vi "picarx.vi"() -> ()   [LabVIEW 2020]
panel:
  in  "Stop Button":bool
  in  "see  up":bool
  in  "see down":bool
  in  "see right":bool
  in  "see left":bool
  in  "backward":bool
  in  "left":bool
  in  "right":bool
  in  "forward":bool
  in  "stop":bool
  in  "say":bool
  in  "Delay Time (s)":dbl=1.0
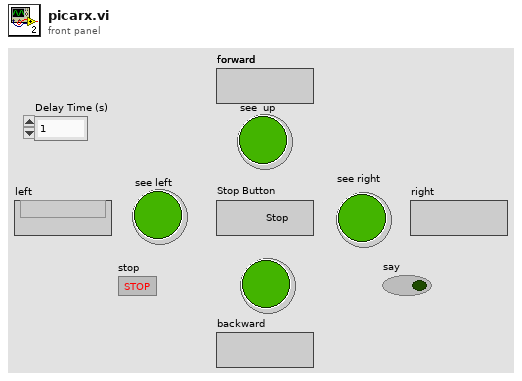
[diagram p1: front panel]
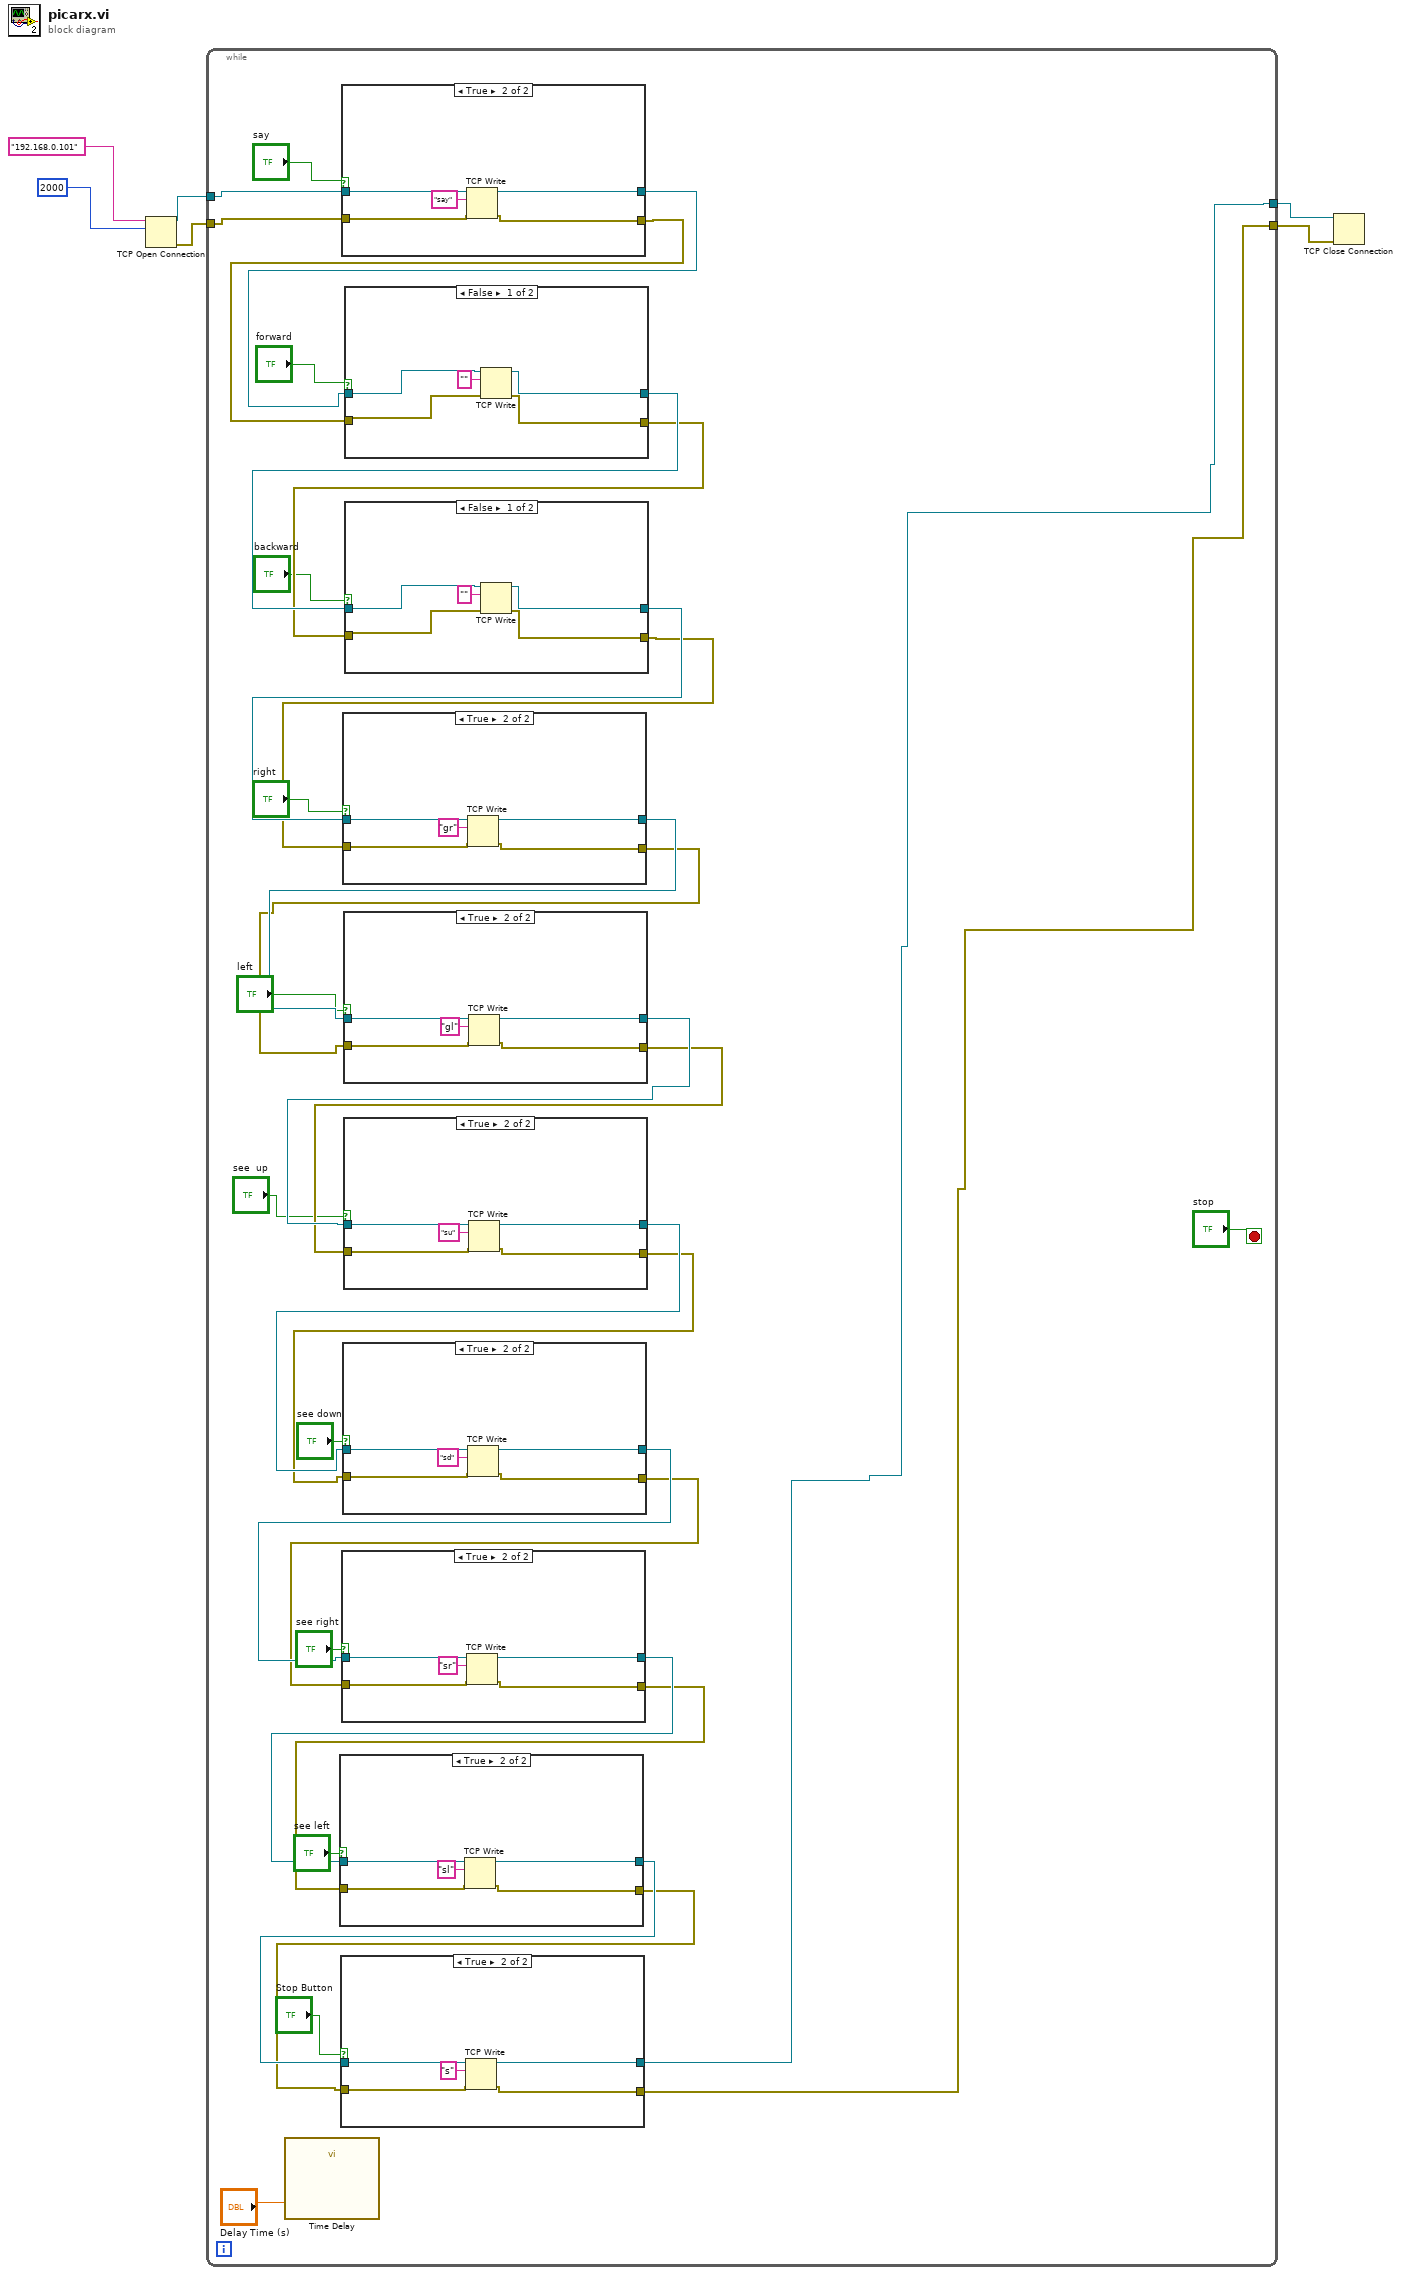
[diagram p0: block diagram]
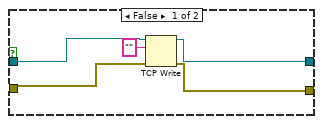
[diagram p2: hidden frame]
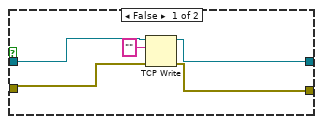
[diagram p3: hidden frame]
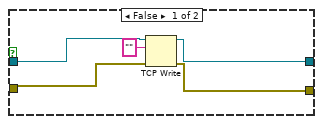
[diagram p4: hidden frame]
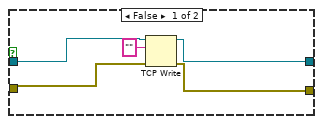
[diagram p5: hidden frame]
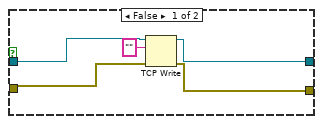
[diagram p6: hidden frame]
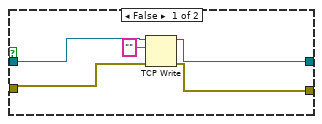
[diagram p7: hidden frame]
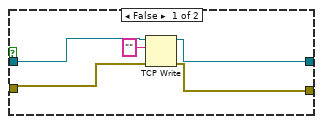
[diagram p8: hidden frame]
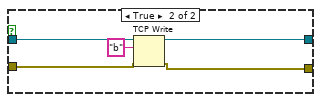
[diagram p9: hidden frame]
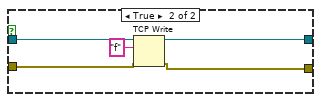
[diagram p10: hidden frame]
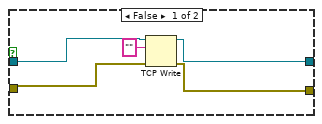
[diagram p11: hidden frame]
diagram:
  n1 = TCP Open Connection(address="192.168.0.101", remote port or service name=u16 2000) -> (connection ID=w5:refnum<k5>, error out=w4:errorcluster)  [unwired: 3 in]
  n2 = while {
    tunnel: [w7] -> w6
    tunnel: w5 -> [w38]
    tunnel: w4 -> [w37]
    tunnel: [w8] -> w1
    stop <- "stop" stop-if-true
    n3 = call "Time Delay"("Delay Time (s)"="Delay Time (s)") -> ()  [unwired: 10 in, 1 out]
    n4 = case shown="True" "say" {
      tunnel: [w133 w140] -> w36
      tunnel: [w132 w139] -> w35
      tunnel: w38 -> [w135 w138]
      tunnel: w37 -> [w134 w137]
      frame False {
        n5 = TCP Write(connection ID=w135, data in="", error in (no error)=w134) -> (connection ID out=w133:refnum<k5>, error out=w132:errorcluster)  [unwired: 1 in, 1 out]
      }
      frame True {
        n6 = TCP Write(connection ID=w138, data in="say", error in (no error)=w137) -> (connection ID out=w140:refnum<k5>, error out=w139:errorcluster)  [unwired: 1 in, 1 out]
      }
    }
    n7 = case shown="False" "forward" {
      tunnel: [w123 w130] -> w34
      tunnel: [w122 w129] -> w33
      tunnel: w36 -> [w125 w128]
      tunnel: w35 -> [w124 w127]
      frame False {
        n8 = TCP Write(connection ID=w125, data in="", error in (no error)=w124) -> (connection ID out=w123:refnum<k5>, error out=w122:errorcluster)  [unwired: 1 in, 1 out]
      }
      frame True {
        n9 = TCP Write(connection ID=w128, data in="f", error in (no error)=w127) -> (connection ID out=w130:refnum<k5>, error out=w129:errorcluster)  [unwired: 1 in, 1 out]
      }
    }
    n10 = case shown="False" "backward" {
      tunnel: [w113 w120] -> w32
      tunnel: [w112 w119] -> w31
      tunnel: w34 -> [w115 w118]
      tunnel: w33 -> [w114 w117]
      frame False {
        n11 = TCP Write(connection ID=w115, data in="", error in (no error)=w114) -> (connection ID out=w113:refnum<k5>, error out=w112:errorcluster)  [unwired: 1 in, 1 out]
      }
      frame True {
        n12 = TCP Write(connection ID=w118, data in="b", error in (no error)=w117) -> (connection ID out=w120:refnum<k5>, error out=w119:errorcluster)  [unwired: 1 in, 1 out]
      }
    }
    n13 = case shown="True" "right" {
      tunnel: [w103 w110] -> w30
      tunnel: [w102 w109] -> w29
      tunnel: w32 -> [w105 w108]
      tunnel: w31 -> [w104 w107]
      frame False {
        n14 = TCP Write(connection ID=w105, data in="", error in (no error)=w104) -> (connection ID out=w103:refnum<k5>, error out=w102:errorcluster)  [unwired: 1 in, 1 out]
      }
      frame True {
        n15 = TCP Write(connection ID=w108, data in="gr", error in (no error)=w107) -> (connection ID out=w110:refnum<k5>, error out=w109:errorcluster)  [unwired: 1 in, 1 out]
      }
    }
    n16 = case shown="True" "left" {
      tunnel: [w93 w100] -> w28
      tunnel: [w92 w99] -> w27
      tunnel: w30 -> [w95 w98]
      tunnel: w29 -> [w94 w97]
      frame False {
        n17 = TCP Write(connection ID=w95, data in="", error in (no error)=w94) -> (connection ID out=w93:refnum<k5>, error out=w92:errorcluster)  [unwired: 1 in, 1 out]
      }
      frame True {
        n18 = TCP Write(connection ID=w98, data in="gl", error in (no error)=w97) -> (connection ID out=w100:refnum<k5>, error out=w99:errorcluster)  [unwired: 1 in, 1 out]
      }
    }
    n19 = case shown="True" "see  up" {
      tunnel: [w83 w90] -> w26
      tunnel: [w82 w89] -> w25
      tunnel: w28 -> [w85 w88]
      tunnel: w27 -> [w84 w87]
      frame False {
        n20 = TCP Write(connection ID=w85, data in="", error in (no error)=w84) -> (connection ID out=w83:refnum<k5>, error out=w82:errorcluster)  [unwired: 1 in, 1 out]
      }
      frame True {
        n21 = TCP Write(connection ID=w88, data in="su", error in (no error)=w87) -> (connection ID out=w90:refnum<k5>, error out=w89:errorcluster)  [unwired: 1 in, 1 out]
      }
    }
    n22 = case shown="True" "see down" {
      tunnel: [w73 w80] -> w24
      tunnel: [w72 w79] -> w23
      tunnel: w26 -> [w75 w78]
      tunnel: w25 -> [w74 w77]
      frame False {
        n23 = TCP Write(connection ID=w75, data in="", error in (no error)=w74) -> (connection ID out=w73:refnum<k5>, error out=w72:errorcluster)  [unwired: 1 in, 1 out]
      }
      frame True {
        n24 = TCP Write(connection ID=w78, data in="sd", error in (no error)=w77) -> (connection ID out=w80:refnum<k5>, error out=w79:errorcluster)  [unwired: 1 in, 1 out]
      }
    }
    n25 = case shown="True" "see right" {
      tunnel: [w63 w70] -> w22
      tunnel: [w62 w69] -> w21
      tunnel: w24 -> [w65 w68]
      tunnel: w23 -> [w64 w67]
      frame False {
        n26 = TCP Write(connection ID=w65, data in="", error in (no error)=w64) -> (connection ID out=w63:refnum<k5>, error out=w62:errorcluster)  [unwired: 1 in, 1 out]
      }
      frame True {
        n27 = TCP Write(connection ID=w68, data in="sr", error in (no error)=w67) -> (connection ID out=w70:refnum<k5>, error out=w69:errorcluster)  [unwired: 1 in, 1 out]
      }
    }
    n28 = case shown="True" "see left" {
      tunnel: [w53 w60] -> w16
      tunnel: [w52 w59] -> w15
      tunnel: w22 -> [w55 w58]
      tunnel: w21 -> [w54 w57]
      frame False {
        n29 = TCP Write(connection ID=w55, data in="", error in (no error)=w54) -> (connection ID out=w53:refnum<k5>, error out=w52:errorcluster)  [unwired: 1 in, 1 out]
      }
      frame True {
        n30 = TCP Write(connection ID=w58, data in="sl", error in (no error)=w57) -> (connection ID out=w60:refnum<k5>, error out=w59:errorcluster)  [unwired: 1 in, 1 out]
      }
    }
    n31 = case shown="True" "Stop Button" {
      tunnel: [w43 w50] -> w8
      tunnel: [w42 w49] -> w7
      tunnel: w16 -> [w45 w48]
      tunnel: w15 -> [w44 w47]
      frame False {
        n32 = TCP Write(connection ID=w45, data in="", error in (no error)=w44) -> (connection ID out=w43:refnum<k5>, error out=w42:errorcluster)  [unwired: 1 in, 1 out]
      }
      frame True {
        n33 = TCP Write(connection ID=w48, data in="s", error in (no error)=w47) -> (connection ID out=w50:refnum<k5>, error out=w49:errorcluster)  [unwired: 1 in, 1 out]
      }
    }
  }
  n34 = TCP Close Connection(connection ID=w1, error in (no error)=w6) -> ()  [unwired: 1 in, 2 out]
